vi "Spawn VI.vi"(6 "State":T1(ring)=enum."Standard", 8 "error in (no error)":errorcluster, 11 "VI reference":refnum<vi>) -> (0 "error out":errorcluster, 2 "Started?":bool)   [LabVIEW 2020]
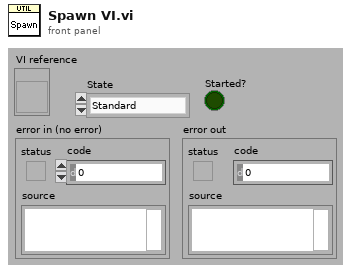
[diagram p1: front panel]
types:
  T1 = enum32{"Invalid", "Standard", "Closed", "Hidden", "Minimized", "Maximized"}
  T2 = enum32{"Bad", "Idle", "Run top level", "Running"}
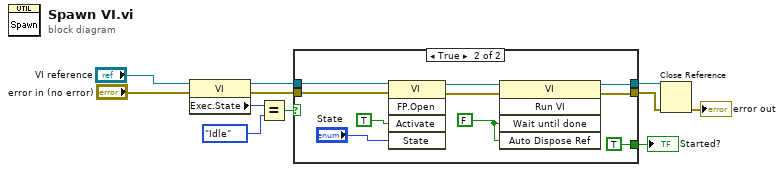
[diagram p0: block diagram]
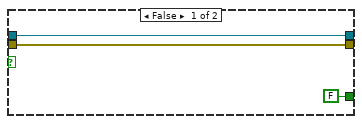
[diagram p2: hidden frame]
diagram:
  n1 = property class="VI"(reference="VI reference", error in="error in (no error)") -> (reference out=w11:refnum<vi>, error out=w10:errorcluster, "Exec.State"=w6:T2)
  n2 = Equal?(x=w6, y=T2."Idle" ("Execution:State")) -> (x = y?=w9:bool)
  n3 = case shown="True" w9 {
    tunnel: w11 -> [w14 w23]
    tunnel: w10 -> [w13 w22]
    tunnel: [w14 w17] -> w8
    tunnel: [w13 w16] -> w7
    tunnel: [FALSE TRUE] -> w1
    frame False {
    }
    frame True {
      w24 = FALSE ("Wait Until Done")
      n4 = invoke class="VI" method="FP.Open"(reference=w23, error in=w22, "Activate"=TRUE ("Activate?"), "State"="State") -> (reference out=w19:refnum<vi>, error out=w18:errorcluster)  [unwired: 1 in, 3 out]
      n5 = invoke class="VI" method="Run VI"(reference=w19, error in=w18, "Wait until done"=w24, "Auto Dispose Ref"=w24) -> (reference out=w17:refnum<vi>, error out=w16:errorcluster)  [unwired: 1 in, 3 out]
    }
  }
  "Started?" <- w1
  n6 = Close Reference(reference=w8, error in (no error)=w7) -> (error out=→"error out":errorcluster)
